vi "HotCoil Test Program.vi"() -> ()   [LabVIEW 2021, in "HotCoil.lvlib"]
uses:
  HotCoil.lvlib
  HotCoil Settings.ctl
panel:
  out "Temp Out":dbl
  out "Running":bool
  out "Connection Error":bool
  in  "stop":bool
  in  "Temp":dbl
  in  "Run":bool
  out "error out":errorcluster
  in  "error in (no error)":errorcluster
  out "HotCoil Settings":T1
  in  "HotCoil Settings":T1
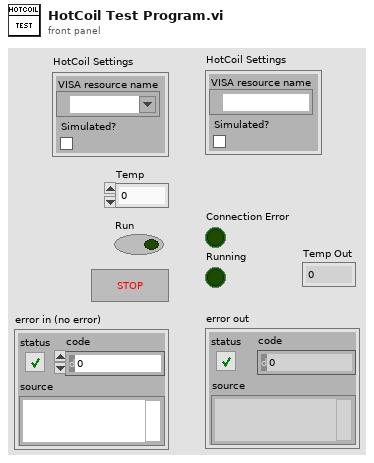
[diagram p1: front panel]
types:
  T1 = typedef "HotCoil.lvlib/HotCoil Settings.ctl" = cluster{"VISA resource name":refnum<visa-resource-name>, "Simulated?":bool}
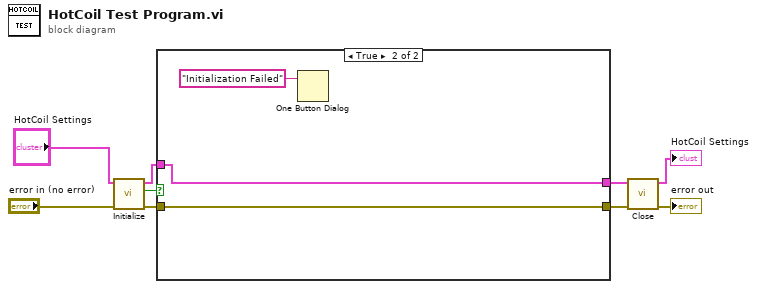
[diagram p0: block diagram]
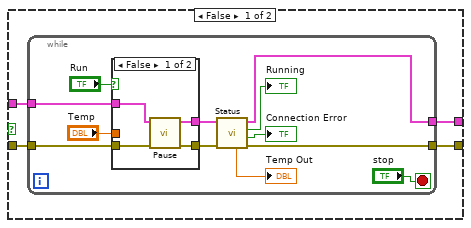
[diagram p2: hidden frame]
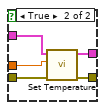
[diagram p3: hidden frame]
diagram:
  n1 = call "Initialize.vi"("error in (no error)"="error in (no error)", "HOTCOIL Settings"="HotCoil Settings") -> ("error out"=w2:errorcluster, "Connection Error"=w1:bool, "HOTCOIL Settings"=w3:T1)  [unwired: 7 in]
  n2 = case shown="True" w1 {
    tunnel: [w13 w36] -> w7
    tunnel: [w12 w35] -> w5
    tunnel: w3 -> [w10 w36]
    tunnel: w2 -> [w11 w35]
    frame False {
      n3 = while {
        tunnel: [w25] -> w13
        tunnel: [w24] -> w12
        tunnel: w11 -> [w22]
        tunnel: w10 -> [w14]
        stop <- "stop" stop-if-true
        n4 = case shown="False" "Run" {
          tunnel: w14 -> [w29 w30]
          tunnel: w22 -> [w28 w34]
          tunnel: [w27 w31] -> w21
          tunnel: [w26 w32] -> w20
          tunnel: "Temp" -> [_ w33]
          frame False {
            n5 = call "Pause.vi"("error in (no error)"=w28, "Julabo FP-50 Settings In"=w29) -> ("error out"=w27:errorcluster, "Julabo FP-50 Settings Out"=w26:T1)  [unwired: 8 in]
          }
          frame True {
            n6 = call "Set Temperature.vi"("error in (no error)"=w34, "Setpoint"=w33, "HotCoil Settings"=w30) -> ("error out"=w31:errorcluster, "HotCoil Settings"=w32:T1)  [unwired: 6 in, 1 out]
          }
        }
        n7 = call "Status.vi"("error in (no error)"=w21, "HotCoil Settings In"=w20) -> ("error out"=w24:errorcluster, "Connection Error"=→"Connection Error":bool, "Running"=→"Running":bool, "HotCoil Settings Out"=w25:T1, "Temp"=→"Temp Out":dbl)  [unwired: 5 in]
      }
    }
    frame True {
      n8 = One Button Dialog(message="Initialization Failed") -> ()  [unwired: 1 in, 1 out]
    }
  }
  n9 = call "Close.vi"("error in (no error)"=w5, "HOTCOIL Settings"=w7) -> ("error out"=→"error out":errorcluster, "HOTCOIL Settings"=→"HotCoil Settings":T1)  [unwired: 8 in]
